vi "RampParaToString.vi"(4 "Mode":T1(ring), 5 "Subfolder Names":string[](array[string]), 6 "Maximum Allowed Current":dbl, 7 "RampSelect":bool[](array[boolean]), 8 "#Points":u32[](array[numeric])=[0, 30, 1, 20] step=1, 9 "WavelengthRamp Parameters":dbl[][](array[numeric]), 10 "TempRamp Parameters":dbl[][](array[numeric]), 11 "FieldRamp Parameters":dbl[][](array[numeric])) -> (0 "Subfolder strings":string, 1 "Wavelength":string, 2 "Temperature":string, 3 "Field":string)   [LabVIEW 2020]
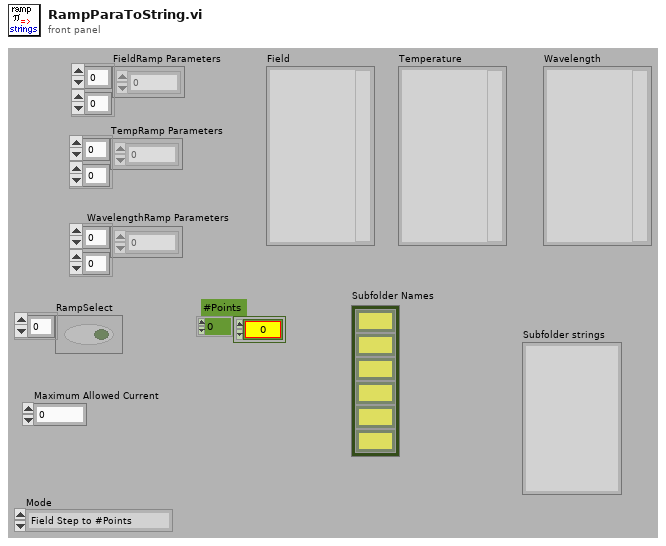
[diagram p1: front panel]
types:
  T1 = enum8{"Field Step to #Points", "#Points to Field Steps"}
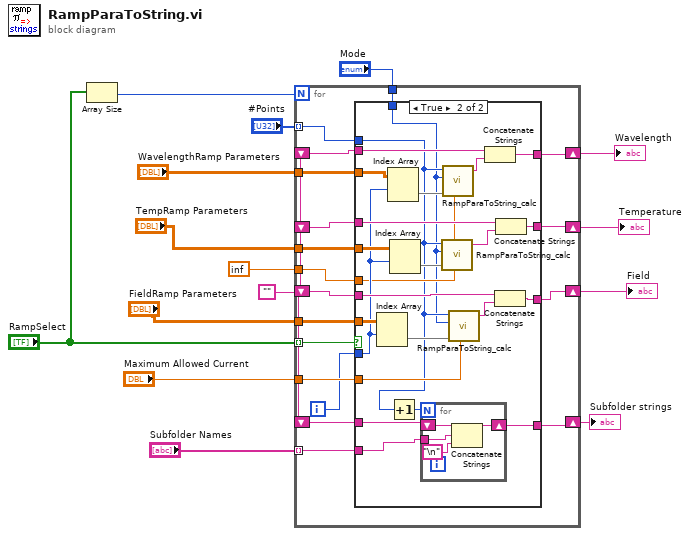
[diagram p0: block diagram]
diagram:
  w4 = ""
  n1 = Array Size(array="RampSelect") -> (size(s)=w1:i32)
  n2 = for {
    N: w1 -> [_]
    tunnel: "RampSelect" -> [w33] mode=indexing
    tunnel: "Maximum Allowed Current" -> [w32]
    tunnel: "FieldRamp Parameters" -> [w31]
    shift-right: [w29] -> w15
    shift-left: w4 -> [w27]
    tunnel: "WavelengthRamp Parameters" -> [w28]
    tunnel: "TempRamp Parameters" -> [w26]
    shift-right: [w25] -> w10
    shift-left: w4 -> [w24]
    shift-right: [w22] -> w9
    shift-left: w4 -> [w23]
    tunnel: inf ("Maximum Allowed Current") -> [w21]
    tunnel: "#Points" -> [w20] mode=indexing
    shift-right: [w19] -> w5
    shift-left: w4 -> [w18]
    tunnel: "Subfolder Names" -> [w17] mode=indexing
    tunnel: "Mode" -> [w16]
    i -> [w30]
    n3 = case shown="True" w33 {
      tunnel: w32 -> [_ w45]
      tunnel: w31 -> [_ w61]
      tunnel: w30 -> [_ w51]
      tunnel: [w35 w60] -> w29
      tunnel: w27 -> [w35 w59]
      tunnel: w24 -> [w37 w55]
      tunnel: w28 -> [_ w54]
      tunnel: w23 -> [w36 w53]
      tunnel: w26 -> [_ w52]
      tunnel: [w37 w50] -> w25
      tunnel: [w36 w49] -> w22
      tunnel: w21 -> [_ w44]
      tunnel: w20 -> [_ w42]
      tunnel: [w34 w41] -> w19
      tunnel: w18 -> [w34 w40]
      tunnel: w17 -> [_ w39]
      tunnel: w16 -> [_ w38]
      frame False {
      }
      frame True {
        n4 = Index Array(array=w61, index (row)=w51) -> (element=w47:dbl[])  [unwired: 1 in]
        n5 = Index Array(array=w54, index (row)=w51) -> (element=w48:dbl[])  [unwired: 1 in]
        n6 = Increment(x=w42) -> (x+1=w43:u32)
        n7 = Index Array(array=w52, index (row)=w51) -> (element=w46:dbl[])  [unwired: 1 in]
        n8 = for {
          N: w43 -> [_]
          shift-right: [w64] -> w41
          shift-left: w40 -> [w62]
          tunnel: w39 -> [w63]
          n9 = Concatenate Strings(w62, w63, "\n") -> (w64:string)
        }
        n10 = call "RampParaToString_calc.vi"("#Points"=w42, "Mode"=w38, "RampParameter"=w46, "Maximum Allowed Current"=w44) -> ("Output String"=w57:string)  [unwired: 1 in, 2 out]
        n11 = call "RampParaToString_calc.vi"("#Points"=w42, "Mode"=w38, "RampParameter"=w48, "Maximum Allowed Current"=w44) -> ("Output String"=w56:string)  [unwired: 1 in, 2 out]
        n12 = call "RampParaToString_calc.vi"("#Points"=w42, "Mode"=w38, "RampParameter"=w47, "Maximum Allowed Current"=w45) -> ("Output String"=w58:string)  [unwired: 1 in, 2 out]
        n13 = Concatenate Strings(w55, w56) -> (w50:string)
        n14 = Concatenate Strings(w59, w58) -> (w60:string)
        n15 = Concatenate Strings(w53, w57) -> (w49:string)
      }
    }
  }
  "Field" <- w15
  "Wavelength" <- w10
  "Temperature" <- w9
  "Subfolder strings" <- w5
